vi "CaseStatement3.vi"() -> ()   [LabVIEW 2014]
panel:
  in  "Operation":T1(ring)
  out "Result":dbl
  in  "B":dbl
  in  "A":dbl
  out "Multiplied":bool
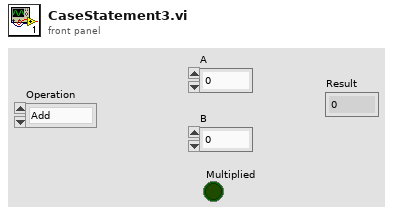
[diagram p1: front panel]
types:
  T1 = enum16{"Add", "Subtract", "Multiply", "Divide", "Log"}
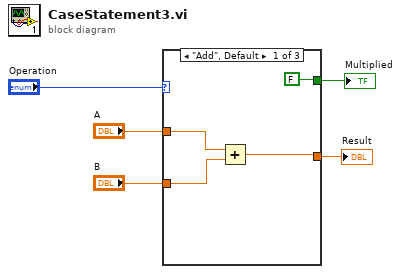
[diagram p0: block diagram]
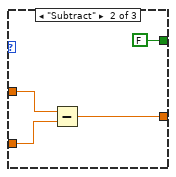
[diagram p2: hidden frame]
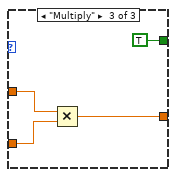
[diagram p3: hidden frame]
diagram:
  n1 = case shown="\"Add\", Default" "Operation" {
    tunnel: "A" -> [w9 w13 w17]
    tunnel: "B" -> [w8 w12 w16]
    tunnel: [w6 w11 w15] -> w3
    tunnel: [FALSE FALSE TRUE] -> w2
    frame "Add", Default {
      n2 = Add(x=w9, y=w8) -> (x+y=w6:dbl)
    }
    frame "Subtract" {
      n3 = Subtract(x=w13, y=w12) -> (x-y=w11:dbl)
    }
    frame "Multiply" {
      n4 = Multiply(x=w17, y=w16) -> (x*y=w15:dbl)
    }
  }
  "Multiplied" <- w2
  "Result" <- w3
